vi "设计性实验-测量电感和直流电阻.vi"() -> ()   [LabVIEW 2021]
panel:
  out "P2":dbl
  out "P1":dbl
  out "F2":dbl
  out "F1":dbl
  out "A2":dbl
  out "A1":dbl
  in  "stop":bool
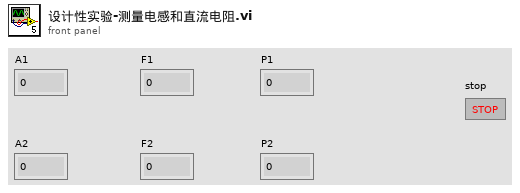
[diagram p1: front panel]
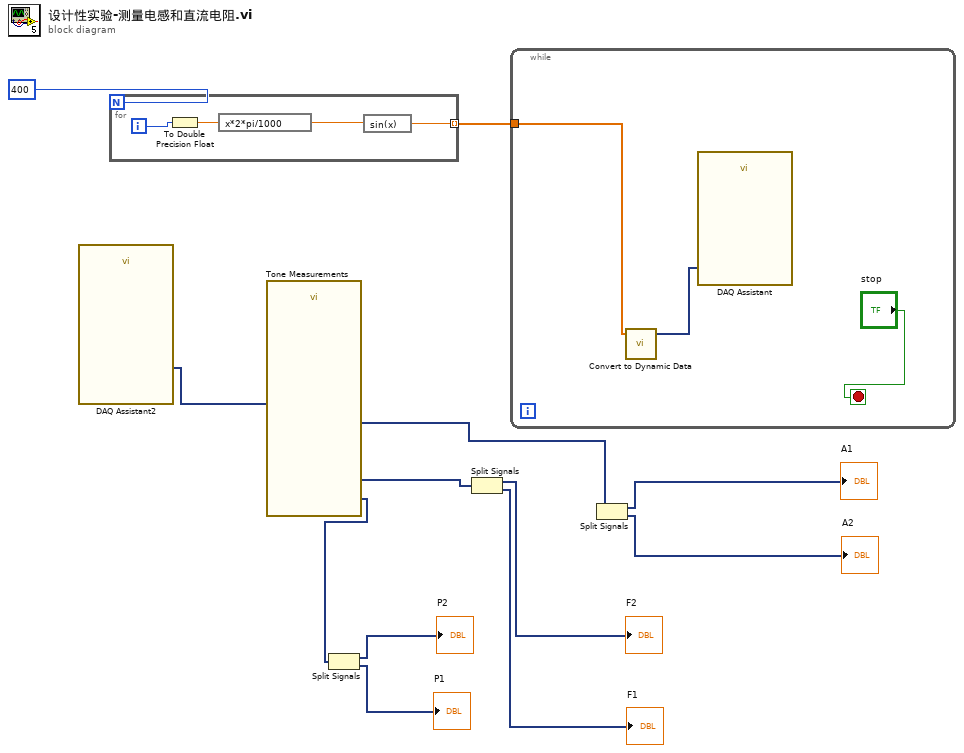
[diagram p0: block diagram]
diagram:
  n1 = call "DAQ Assistant2"() -> ("data"=w10:dynamicdata)  [unwired: 17 in, 2 out]
  n2 = for {
    N: 400 -> [_]
    tunnel: [w13] -> w11 mode=indexing
    i -> [w16]
    n3 = To Double Precision Float(number=w16) -> (double precision float=w15:dbl)
    n4 = expression code="x*2*pi/1000"(w15) -> (w14:dbl)
    n5 = expression code="sin(x)"(w14) -> (w13:dbl)
  }
  n6 = call "Tone Measurements"("Signals"=w10) -> ("Phase"=w1:dynamicdata, "Frequency"=w6:dynamicdata, "Amplitude"=w9:dynamicdata)  [unwired: 7 in, 1 out]
  n7 = Split Signals(w1) -> (→"P2":dynamicdata, →"P1":dynamicdata)  [unwired: 2 in]
  n8 = Split Signals(w6) -> (→"F2":dynamicdata, →"F1":dynamicdata)  [unwired: 2 in]
  n9 = while {
    tunnel: w11 -> [w17]
    stop <- "stop" stop-if-true
    n10 = call "Convert to Dynamic Data"("Array"=w17) -> ("Dynamic Data Type"=w19:dynamicdata)  [unwired: 3 in]
    n11 = call "DAQ Assistant"("data"=w19) -> ()  [unwired: 16 in, 3 out]
  }
  n12 = Split Signals(w9) -> (→"A1":dynamicdata, →"A2":dynamicdata)  [unwired: 2 in]
